vi "ManualHoodControl.vi"(8 "Button 6":bool, 9 "Button 7":bool, 10 "Tilt Value":bool, 11 "MotorControlDevRef":T1={"DeviceStatus"={"status"=FALSE, "code"=0, "source"=""}, "Type"=enum."PWM", "PWM"={"Digital Module"=enum."Digital Module 1", "PWM Channel"=enum."Invalid", "DeadBand"={"Name"="", "maxPositivePwm"=0, "minPositivePwm"=0, "centerPwm"=0, "maxNegativePwm"=0, "minNegativePwm"=0, "angularRange"=0}}, "CAN"={"Device Number"=0, "Control Mode"=enum."Percent VBus", "Semaphore"=refnum, "Max Vout"=12.0}, "Invert"=FALSE, "TransformRef"=refnum, "InvTransformRef"=refnum}) -> ()   [LabVIEW 2011]
uses:
  <vilib>/Rock Robotics/WPI/MotorControl/WPI_MotorControlDeviceRef.ctl
  <vilib>/Rock Robotics/SystemInterfaces/Typedef/FPGA_TypedefDigitalModule.ctl
  <vilib>/Rock Robotics/SystemInterfaces/DIO/FPGA_DIOPWMChannel.ctl
  <vilib>/Rock Robotics/WPI/PWM/WPI_PWMDeadband.ctl
  <vilib>/Rock Robotics/WPI/CAN/Jaguar/SubVIs/WPI_CANJaguar_ControlMode.ctl
  <vilib>/Rock Robotics/WPI/PWM/WPI_PWMTransform_ConPane.ctl
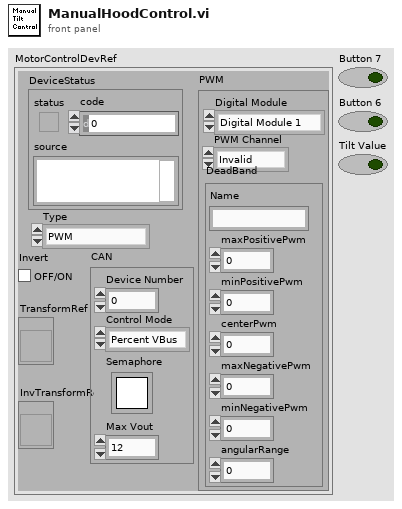
[diagram p1: front panel]
types:
  T1 = typedef "WPI_MotorControlDeviceRef.ctl" = cluster{"DeviceStatus":errorcluster, "Type":enum16{"PWM", "CAN"}, "PWM":cluster{"Digital Module":T2, "PWM Channel":T3, "DeadBand":T4}, "CAN":cluster{"Device Number":u8, "Control Mode":T5, "Semaphore":T6, "Max Vout":dbl}, "Invert":bool, "TransformRef":T7, "InvTransformRef":T7}
  T2 = typedef "FPGA_TypedefDigitalModule.ctl" = enum16{"Digital Module 1", "Digital Module 2"}
  T3 = typedef "FPGA_DIOPWMChannel.ctl" = enum8{"PWM 1", "PWM 2", "PWM 3", "PWM 4", "PWM 5", "PWM 6", "PWM 7", "PWM 8", "PWM 9", "PWM 10", "Invalid"}
  T4 = typedef "WPI_PWMDeadband.ctl" = cluster{"Name":string, "maxPositivePwm":i32, "minPositivePwm":i32, "centerPwm":i32, "maxNegativePwm":i32, "minNegativePwm":i32, "angularRange":u16}
  T5 = typedef "WPI_CANJaguar_ControlMode.ctl" = enum8{"Percent VBus", "Current", "Speed", "Position", "Voltage"}
  T6 = typedef "Semaphore RefNum" = refnum<k1>
  T7 = typedef "WPI_PWMTransform_ConPane.ctl" = refnum<vi>
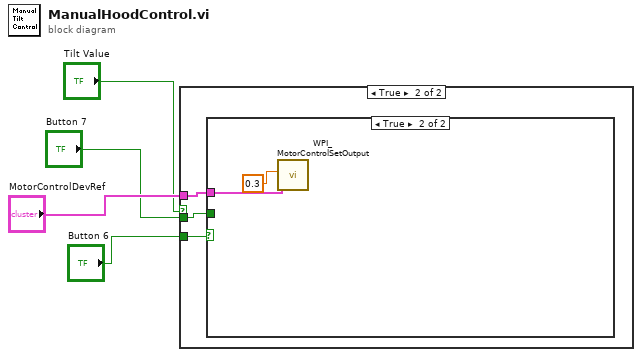
[diagram p0: block diagram]
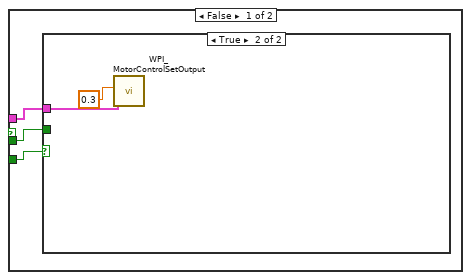
[diagram p2: hidden frame]
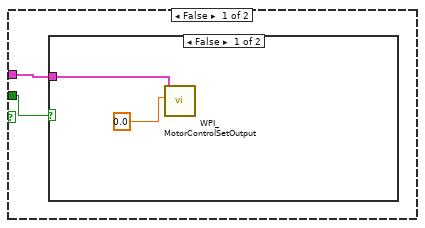
[diagram p3: hidden frame]
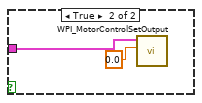
[diagram p4: hidden frame]
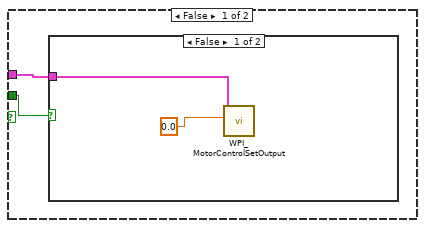
[diagram p5: hidden frame]
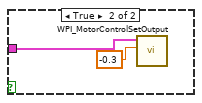
[diagram p6: hidden frame]
diagram:
  n1 = case shown="True" "Tilt Value" {
    tunnel: "Button 6" -> [w5 w18]
    tunnel: "Button 7" -> [w6 w17]
    tunnel: "MotorControlDevRef" -> [w7 w16]
    frame False {
      n2 = case shown="True" w5 {
        tunnel: w6 -> [w9 _]
        tunnel: w7 -> [w8 w14]
        frame False {
          n3 = case shown="False" w9 {
            tunnel: w8 -> [w10 w12]
            frame False {
              n4 = call <vilib>:"WPI_MotorControlSetOutput.vi"("Output"=0.0, "MotorControlDevRef"=w10) -> ()  [unwired: 8 in, 2 out]
            }
            frame True {
              n5 = call <vilib>:"WPI_MotorControlSetOutput.vi"("Output"=0.0, "MotorControlDevRef"=w12) -> ()  [unwired: 8 in, 2 out]
            }
          }
        }
        frame True {
          n6 = call <vilib>:"WPI_MotorControlSetOutput.vi"("Output"=0.3, "MotorControlDevRef"=w14) -> ()  [unwired: 8 in, 2 out]
        }
      }
    }
    frame True {
      n7 = case shown="True" w18 {
        tunnel: w17 -> [w20 _]
        tunnel: w16 -> [w19 w25]
        frame False {
          n8 = case shown="False" w20 {
            tunnel: w19 -> [w21 w23]
            frame False {
              n9 = call <vilib>:"WPI_MotorControlSetOutput.vi"("Output"=0.0, "MotorControlDevRef"=w21) -> ()  [unwired: 8 in, 2 out]
            }
            frame True {
              n10 = call <vilib>:"WPI_MotorControlSetOutput.vi"("Output"=-0.3, "MotorControlDevRef"=w23) -> ()  [unwired: 8 in, 2 out]
            }
          }
        }
        frame True {
          n11 = call <vilib>:"WPI_MotorControlSetOutput.vi"("Output"=0.3, "MotorControlDevRef"=w25) -> ()  [unwired: 8 in, 2 out]
        }
      }
    }
  }
